vi "Set Format.vi"(8 "error in (no error)":errorcluster caption="错误输入（无错误）", 10 "Format":string, 11 "SpecificString 输入":refnum<class "SpecificString.lvclass">) -> (0 "error out":errorcluster caption="错误输出", 3 "SpecificString 输出":refnum<class "SpecificString.lvclass">)   [LabVIEW 2018, in "SpecificString.lvclass"]
uses:
  SpecificString.lvclass
  SpecificString.lvclass/SpecificString.ctl
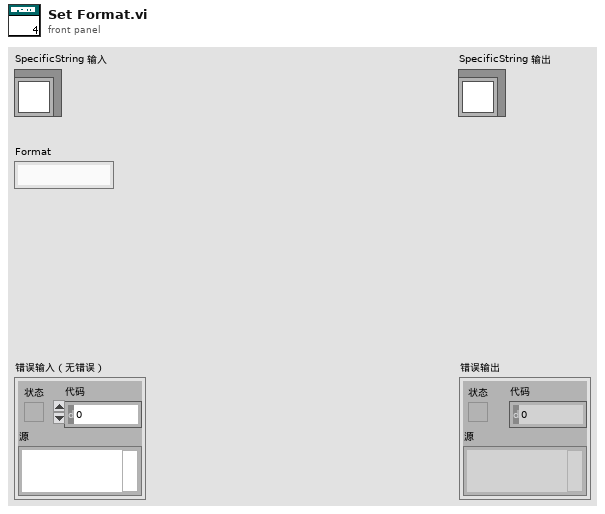
[diagram p1: front panel]
types:
  T1 = typedef "SpecificString.lvclass/State Data.ctl" = cluster{"Format":string, "Correct Color":u32, "Error Color":u32}
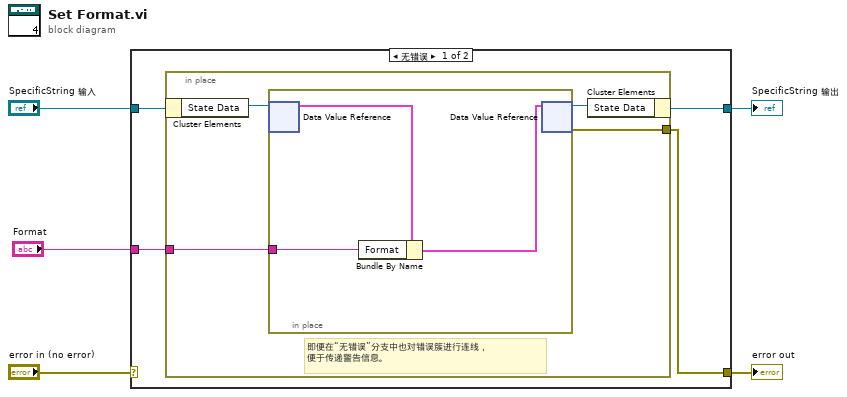
[diagram p0: block diagram]
diagram:
  n1 = case shown="无错误" "error in (no error)" {
    selector: "error in (no error)" -> [_ w18]
    tunnel: [w7 w18] -> w4
    tunnel: [w8 w17] -> w2
    tunnel: "SpecificString 输入" -> [w9 w17]
    tunnel: "Format" -> [w6 _]
    frame No Error {
      n2 = in-place {
        in-place-border: [w11] -> w7
        in-place-border: w6 -> [w10]
        # "即便在“无错误”分支中也对错误簇进行连线，\n便于传递警告信息。"
        n3 = in-place-cluster #1(w9) -> ("State Data"=w13:refnum<data-value>)
        n4 = in-place {
          in-place-border: w10 -> [w14]
          n5 = in-place-dvr #2(w13) -> (w16:T1)  [unwired: 1 out]
          n6 = Bundle By Name(cluster=w16, "Format"=w14) -> (w15:T1)
          n7 = in-place-dvr #2(w15) -> (w12:refnum<data-value>, w11:errorcluster)
        }
        n8 = in-place-cluster #1("State Data"=w12) -> (w8:refnum<class "SpecificString.lvclass">)
      }
    }
    frame Error {
    }
  }
  "error out" <- w4
  "SpecificString 输出" <- w2
